vi "Sorted Particle Report.vi"(3 "Min Area Size %":dbl, 4 "Particle Count Limit":i32=2147483647, 5 "Pixel Measurements":T2[](array[typedef])=[35, 4, 5, 6, 7] items=["Center of Mass X", "Center of Mass Y", "First Pixel X", "First Pixel Y", "Bounding Rect Left", "Bounding Rect Top", "Bounding Rect Right", "Bounding Rect Bottom", "Max Feret Diameter Start X", "Max Feret Diameter Start Y", "Max Feret Diameter End X", "Max Feret Diameter End Y", "Max Horiz. Segment Length Left", "Max Horiz. Segment Length Right", "Max Horiz. Segment Length Row", "-", "Bounding Rect Width", "Bounding Rect Height", "Bounding Rect Diagonal", "Perimeter", "Convex Hull Perimeter", "Holes' Perimeter", "Max Feret Diameter", "Equivalent Ellipse Major Axis", "Equivalent Ellipse Minor Axis", "Equivalent Ellipse Minor Axis (Feret)", "Equivalent Rect Long Side", "Equivalent Rect Short Side", "Equivalent Rect Diagonal", "Equivalent Rect Short Side (Feret)", "Average Horiz. Segment Length", "Average Vert. Segment Length", "Hydraulic Radius", "Waddel Disk Diameter", "-", "Area", "Holes' Area", "Particle & Holes' Area", "Convex Hull Area", "Image Area", "-", "Number of Holes", "Number of Horiz. Segments", "Number of Vert. Segments", "-", "Orientation", "Max Feret Diameter Orientation", "-", "% Area/Image Area", "% Area/(Particle & Holes' Area)", "Ratio of Equivalent Ellipse Axes", "Ratio of Equivalent Rect Sides", "-", "Elongation Factor", "Compactness Factor", "Heywood Circularity Factor", "Type Factor", "-", "Sum X", "Sum Y", "Sum XX", "Sum XY", "Sum YY", "Sum XXX", "Sum XXY", "Sum XYY", "Sum YYY", "-", "Moment of Inertia XX", "Moment of Inertia XY", "Moment of Inertia YY", "Moment of Inertia XXX", "Moment of Inertia XXY", "Moment of Inertia XYY", "Moment of Inertia YYY", "Norm. Moment of Inertia XX", "Norm. Moment of Inertia XY", "Norm. Moment of Inertia YY", "Norm. Moment of Inertia XXX", "Norm. Moment of Inertia XXY", "Norm. Moment of Inertia XYY", "Norm. Moment of Inertia YYY", "Hu Moment 1", "Hu Moment 2", "Hu Moment 3", "Hu Moment 4", "Hu Moment 5", "Hu Moment 6", "Hu Moment 7"], 6 "Image in":T3) -> (0 "limits":T1, 1 "Sorted Data":dbl[][](array[numeric]), 2 "Particles":i32)   [LabVIEW 2019]
doc: "Returns the requested measurements of a binary image sorted by the first parameter (often size), and limiting the rows in the 2D array by count and by size. Pass infinity to count to avoid a limit. Pass zero to size to avoid a limit."
uses:
  <vilib>/vision/Image Controls.llb/IMAQ Image.ctl
  <vilib>/vision/NI_Vision_Development_Module.lvlib
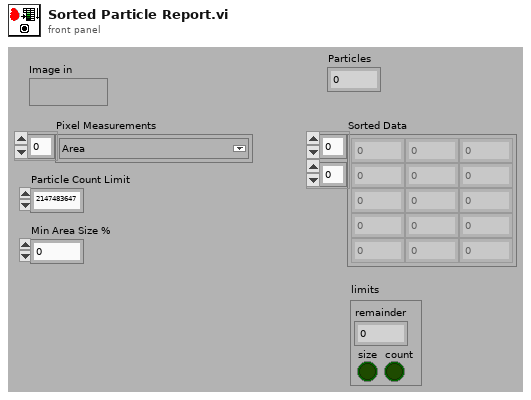
[diagram p1: front panel]
types:
  T1 = cluster{"remainder":i32, "size":bool, "count":bool}
  T2 = typedef "Particle Parameters" = i32
  T3 = typedef "IMAQ Image.ctl" = refnum<image>
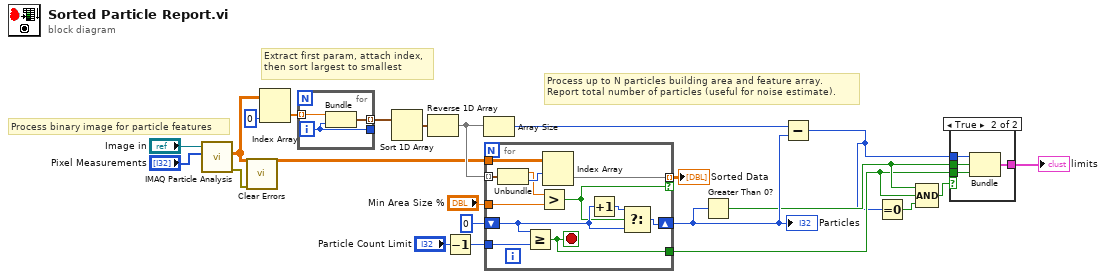
[diagram p0: block diagram]
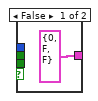
[diagram p2: hidden frame]
diagram:
  # "Process up to N particles building area and feature array.\nReport total number of particles (useful for noise estimate)."
  # "Process binary image for particle features"
  # "Extract first param, attach index,\nthen sort largest to smallest"
  n1 = call "IMAQ Particle Analysis"("Pixel Measurements"="Pixel Measurements", "Image"="Image in") -> ("error out"=w13:errorcluster, "Particle Measurements (Pixels)"=w11:dbl[][])  [unwired: 3 in, 5 out]
  n2 = call <vilib>:"Clear Errors.vi"("error in (no error)"=w13) -> ()  [unwired: 5 in, 2 out]
  n3 = Index Array(array=w11, index (col)=0 ("disabled index (col)")) -> (element=w19:dbl[])  [unwired: 1 in]
  n4 = for {
    tunnel: w19 -> [w25] mode=indexing
    tunnel: [w24] -> w20 mode=indexing
    tunnel: [w23] -> _
    i -> [w23]
    n5 = Bundle("Numeric"=w25, w23) -> (w24:cluster{"Numeric":dbl, i32})  [unwired: 1 out]
  }
  n6 = Sort 1D Array(array=w20) -> (sorted array=w21:cluster{"Numeric":dbl, i32}[])
  n7 = Reverse 1D Array(array=w21) -> (reversed array=w12:cluster{"Numeric":dbl, i32}[])
  n8 = Decrement(x="Particle Count Limit") -> (x-1=w9:i32)
  n9 = Array Size(array=w12) -> (size(s)=w15:i32)
  n10 = for {
    tunnel: w11 -> [w36]
    tunnel: w12 -> [w35] mode=indexing
    tunnel: w9 -> [w34]
    tunnel: "Min Area Size %" -> [w32]
    tunnel: [w30] -> w4
    tunnel: [w31] -> w8 mode=indexing if=w26
    shift-right: [w29] -> w6
    shift-left: 0 -> [w27]
    stop <- w30 stop-if-true
    n11 = Unbundle(w35) -> ("Numeric"=w33:dbl, w37:i32)
    n12 = Greater Or Equal?(x=w27, y=w34) -> (x >= y?=w30:bool)
    n13 = Greater?(x=w33, y=w32) -> (0:w26:bool)
    n14 = Index Array(array=w36, index (row)=w37) -> (element=w31:dbl[])  [unwired: 1 in]
    n15 = Increment(x=w27) -> (x+1=w28:i32)
    n16 = Select(t=w28, s=w26, f=w27) -> (s? t:f=w29:i32)
  }
  "Particles" <- w6
  "Sorted Data" <- w8
  n17 = Greater Than 0?(x=w6) -> (x > 0?=w5:bool)
  n18 = Subtract(x=w15, y=w6) -> (x-y=w2:i32)
  n19 = Equal To 0?(x=w2) -> (x = 0?=w1:bool)
  n20 = Compound Arithmetic op=AND(w5, w4, w1) -> (w3:bool)
  n21 = case shown="True" w3 {
    tunnel: w2 -> [_ w42]
    tunnel: [cluster{i32, bool, bool} {0, FALSE, FALSE} w41] -> w14
    tunnel: w5 -> [_ w40]
    tunnel: w4 -> [_ w39]
    frame False {
    }
    frame True {
      n22 = Bundle(w42, w40, w39) -> (w41:cluster{i32, bool, bool})  [unwired: 1 in]
    }
  }
  "limits" <- w14
